vi "Forward Pass Array (RNN).vi"(0 "inputs":i32[](array[numeric])=[1], 1 "dimension":i32=3, 2 "hprev":T1=[[0.0], [0.0]] format="%_8f", 3 "params":T2={"Wxh"=[[0.578129, 2.569937, -0.0219857], [-2.46959, 0.027262, 2.449614362]], "Whh"=[[-1.3996, 0.961745], [0.364566, -0.477064]], "bh"=[[0.535351], [-1.985987]], "Why"=[[-0.658616, 0.764692], [-1.7789986, 0.388036], [-0.130912, -0.333988]], "by"=[[-0.528417], [-0.44032], [-0.8844819]]} {"Wxh" format="%_8f"; "Whh" format="%_8f"; "bh" format="%_8f"; "Why" format="%_8f"; "by" format="%_8f"}) -> (7 "xs":dbl[][][](array[numeric])=[[[0.0], [1.0], [0.0]]], 8 "hs":dbl[][][](array[numeric])=[[[0.0], [0.0]], [[0.9959918876590693], [-0.9609924209716473]]] format="%_8f", 9 "ps":dbl[][][](array[numeric])=[[[0.2032853269546711], [0.10445737822381787], [0.6922572948215111]]] format="%_8f", 10 "h_latest":T1=[[0.9959918876590693], [-0.9609924209716473]] format="%_8f")   [LabVIEW 2014]
uses:
  <vilib>/Analysis/Matrix/Datatypes/RealMatrix.ctl
  <vilib>/Analysis/Matrix/NI_Matrix.lvlib
panel:
  # "INPUT"
  # "OUTPUT"
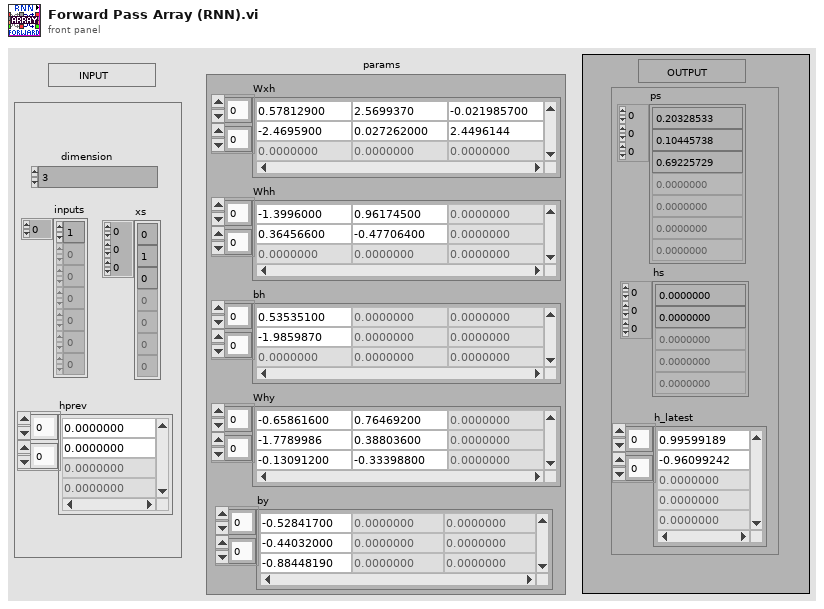
[diagram p1: front panel]
types:
  T1 = typedef "NI_Matrix.lvlib/RealMatrix.ctl" = dbl[][]
  T2 = cluster{"Wxh":T1, "Whh":T1, "bh":T1, "Why":T1, "by":T1}
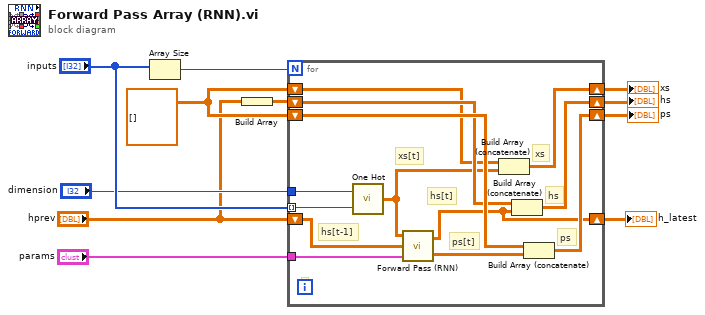
[diagram p0: block diagram]
diagram:
  w7 = dbl[][][] []
  n1 = Array Size(array="inputs") -> (size(s)=w11:i32)
  n2 = Build Array("hprev") -> (w1:dbl[][][])
  n3 = for {
    N: w11 -> [_]
    shift-right: [w12] -> w3
    shift-left: "hprev" -> [w13]
    tunnel: "params" -> [w24]
    tunnel: "dimension" -> [w22]
    tunnel: "inputs" -> [w23] mode=indexing
    shift-right: [w20] -> w10
    shift-left: w7 -> [w17]
    shift-right: [w19] -> w9
    shift-left: w1 -> [w16]
    shift-right: [w18] -> w8
    shift-left: w7 -> [w15]
    # "t"
    # "hs[t-1]"
    # "xs[t]"
    # "hs[t]"
    # "ps[t]"
    # "ps"
    # "hs"
    # "xs"
    n4 = call "One Hot.vi"("hot index"=w23, "length"=w22) -> ("One hot vector"=w14:T1)
    n5 = call "Forward Pass (RNN).vi"("params"=w24, "h[t-1]"=w13, "x[t]"=w14) -> ("p[t]"=w21:T1, "h[t]"=w12:T1)
    n6 = Build Array (concatenate)(w15, w14) -> (w18:dbl[][][])
    n7 = Build Array (concatenate)(w16, w12) -> (w19:dbl[][][])
    n8 = Build Array (concatenate)(w17, w21) -> (w20:dbl[][][])
  }
  "ps" <- w10
  "hs" <- w9
  "xs" <- w8
  "h_latest" <- w3
